vi "Project Run All Tests.vi"(8 "error in (no error)":errorcluster, 11 "VI Tester reference":refnum<vi>) -> (0 "error out":errorcluster)   [LabVIEW 2011, in "VI Tester Project API.lvlib"]
uses:
  VI Tester Project API.lvlib
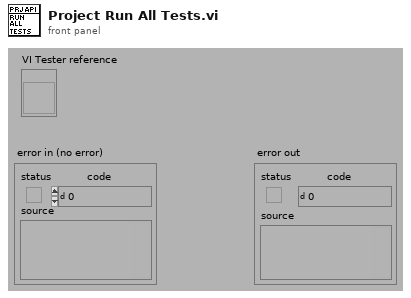
[diagram p1: front panel]
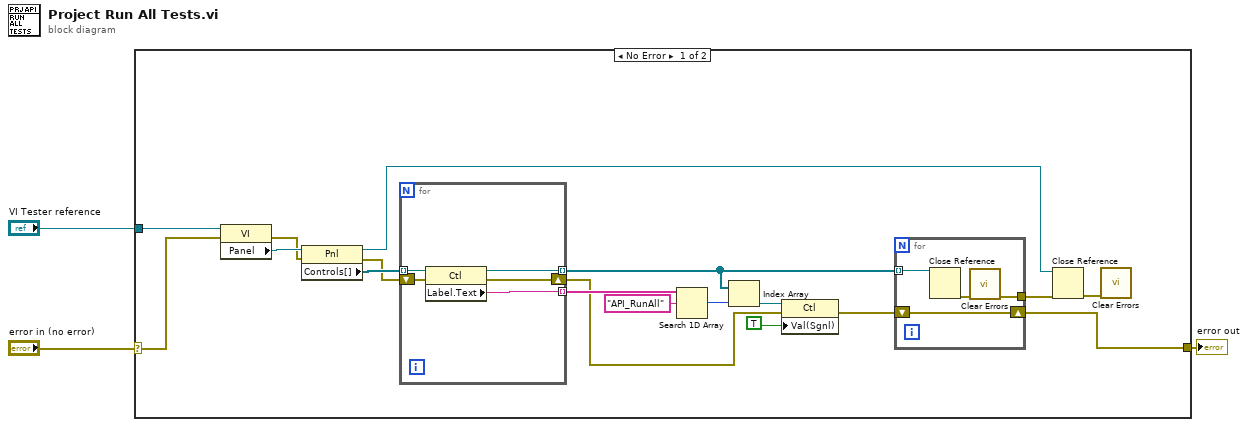
[diagram p0: block diagram]
diagram:
  n1 = case shown="No Error" "error in (no error)" {
    selector: "error in (no error)" -> [w5 w31]
    tunnel: [w9 w31] -> w3
    tunnel: "VI Tester reference" -> [w6 _]
    frame No Error {
      n2 = property class="VI"(reference=w6, error in=w5) -> (error out=w20:errorcluster, "Panel"=w21:refnum<vi>)  [unwired: 1 out]
      n3 = property class="Pnl"(reference=w21, error in=w20) -> (reference out=w8:refnum<vi>, error out=w18:errorcluster, "Controls[]"=w19:refnum<vi>[])
      n4 = for {
        tunnel: w19 -> [w30] mode=indexing
        tunnel: [w29] -> w17 mode=indexing
        shift-right: [w27] -> w11
        shift-left: w18 -> [w28]
        tunnel: [w26] -> w12 mode=indexing
        n5 = property class="Ctl"(reference=w30, error in=w28) -> (reference out=w26:refnum<vi>, error out=w27:errorcluster, "Label.Text"=w29:string)
      }
      n6 = Search 1D Array(1D array=w17, element="API_RunAll") -> (index of element=w15:i32)  [unwired: 1 in]
      n7 = Index Array(array=w12, index=w15) -> (element=w14:refnum<vi>)
      n8 = property class="Ctl"(reference=w14, error in=w11, "Val(Sgnl)"=TRUE) -> (error out=w10:errorcluster)  [unwired: 1 out]
      n9 = for {
        tunnel: w12 -> [w25] mode=indexing
        shift-right: [w24] -> w9
        shift-left: w10 -> [w24]
        tunnel: [w22] -> w7
        n10 = Close Reference(reference=w25) -> (error out=w23:errorcluster)  [unwired: 1 in]
        n11 = call <vilib>:"Clear Errors.vi"("error in (no error)"=w23) -> ("error out"=w22:errorcluster)  [unwired: 6 in]
      }
      n12 = Close Reference(reference=w8, error in (no error)=w7) -> (error out=w4:errorcluster)
      n13 = call <vilib>:"Clear Errors.vi"("error in (no error)"=w4) -> ()  [unwired: 6 in, 1 out]
    }
    frame Error {
    }
  }
  "error out" <- w3
